vi "dfd_Check Log Spaced Plot Settings.vi"(6 "fs [Hz] in":dbl=-1.0 format="%.2f", 8 "error in (no error)":errorcluster, 10 "filter fs[Hz]":dbl, 11 "plot settings":T1={"# freq bins"=-1, "low frequency [Hz]"=0.01, "high frequency [Hz]"=0.5}) -> (0 "error out":errorcluster, 3 "plot settings out":T1={"# freq bins"=-1, "low frequency [Hz]"=0.01, "high frequency [Hz]"=0.5}, 4 "fs out [Hz]":dbl)   [LabVIEW 2017, in "NI_DigFilterLicensed.lvlib"]
uses:
  <vilib>/addons/Digital Filter Design/NI_DigFilterLicensed.lvlib
  <vilib>/addons/Digital Filter Design/_Objects.llb/DFD Plot Settings.ctl
  <vilib>/addons/Digital Filter Design/_Misc.llb/dfd_Error Handlers (Single).vi
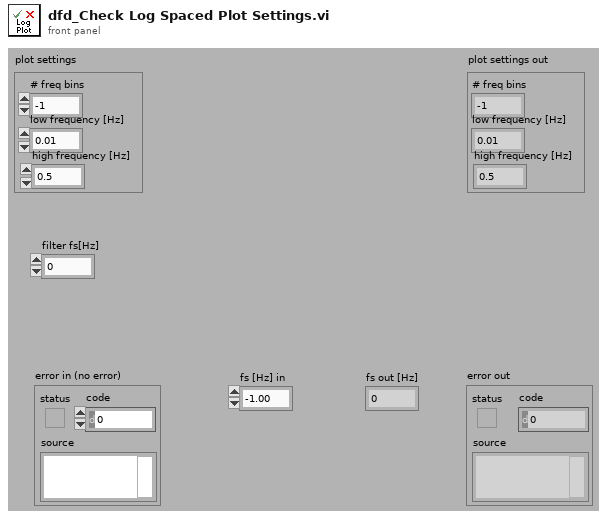
[diagram p1: front panel]
types:
  T1 = typedef "NI_DigFilterLicensed.lvlib/DFD Plot Settings.ctl" = cluster{"# freq bins":i32, "low frequency [Hz]":dbl, "high frequency [Hz]":dbl}
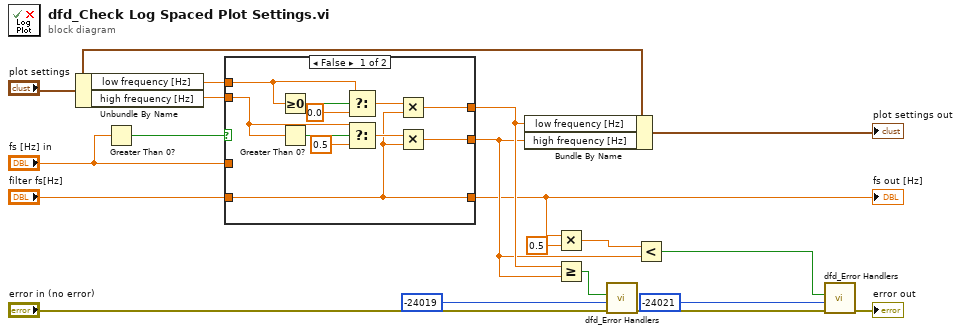
[diagram p0: block diagram]
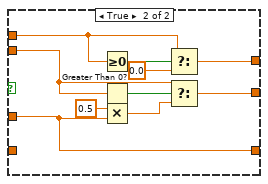
[diagram p2: hidden frame]
diagram:
  n1 = Unbundle By Name("plot settings") -> ("low frequency [Hz]"=w18:dbl, "high frequency [Hz]"=w17:dbl)
  n2 = Greater Than 0?(x="fs [Hz] in") -> (x > 0?=w19:bool)
  n3 = case shown="False" w19 {
    tunnel: "fs [Hz] in" -> [_ w31]
    tunnel: w18 -> [w27 w39]
    tunnel: [w22 w37] -> w10
    tunnel: w17 -> [w26 w35]
    tunnel: [w21 w32] -> w9
    tunnel: [w20 w31] -> w3
    tunnel: "filter fs[Hz]" -> [w20 _]
    frame False {
      n4 = Greater Or Equal To 0?(x=w27) -> (x >= 0?=w30:bool)
      n5 = Greater Than 0?(x=w26) -> (x > 0?=w28:bool)
      n6 = Select(t=w27, s=w30, f=0.0) -> (s? t:f=w24:dbl)
      n7 = Select(t=w26, s=w28, f=0.5) -> (s? t:f=w23:dbl)
      n8 = Multiply(x=w24, y=w20) -> (x*y=w22:dbl)
      n9 = Multiply(x=w23, y=w20) -> (x*y=w21:dbl)
    }
    frame True {
      n10 = Greater Or Equal To 0?(x=w39) -> (x >= 0?=w40:bool)
      n11 = Greater Than 0?(x=w35) -> (x > 0?=w36:bool)
      n12 = Multiply(x=0.5 ("f"), y=w31) -> (x*y=w33:dbl)
      n13 = Select(t=w39, s=w40, f=0.0) -> (s? t:f=w37:dbl)
      n14 = Select(t=w35, s=w36, f=w33) -> (s? t:f=w32:dbl)
    }
  }
  "fs out [Hz]" <- w3
  n15 = Bundle By Name(cluster="plot settings", "low frequency [Hz]"=w10, "high frequency [Hz]"=w9) -> (→"plot settings out":T1)
  n16 = Multiply(x=w3, y=0.5) -> (x*y=w14:dbl)
  n17 = Greater Or Equal?(x=w10, y=w9) -> (x >= y?=w13:bool)
  n18 = call-poly <vilib>:"dfd_Error Handlers.vi"("error in (no error)"="error in (no error)", "error code"=-24019 ("ERR_FREQ_NOT_ASCENDING"), "condition failed?"=w13) -> ("error out"=w12:errorcluster)  [unwired: 8 out]
  n19 = Less?(x=w14, y=w9) -> (x < y?=w1:bool)
  n20 = call-poly <vilib>:"dfd_Error Handlers.vi"("error in (no error)"=w12, "error code"=-24021 ("ERR_FREQ_RANGE_WRONG"), "condition failed?"=w1) -> ("error out"=→"error out":errorcluster)  [unwired: 8 out]
